vi "ad float to sample.vi"(6 "dbl":sgl, 7 "sample":u32, 8 "error in (no error)":errorcluster, 9 "range":i32, 10 "cha":i32, 11 "adh":i32) -> (0 "error out":errorcluster, 3 "function return":i32, 5 "sample out":u32)   [LabVIEW 2021, in "libad4.lvlib"]
doc: "ad_float_to_sample (int32_t adh, int32_t cha, int32_t range, float dbl, uint32_t *sample);\n\nConverts a float value into a sample value."
uses:
  <userlib>/libad4/libad4.lvlib
  <userlib>/libad4/libad4.dll
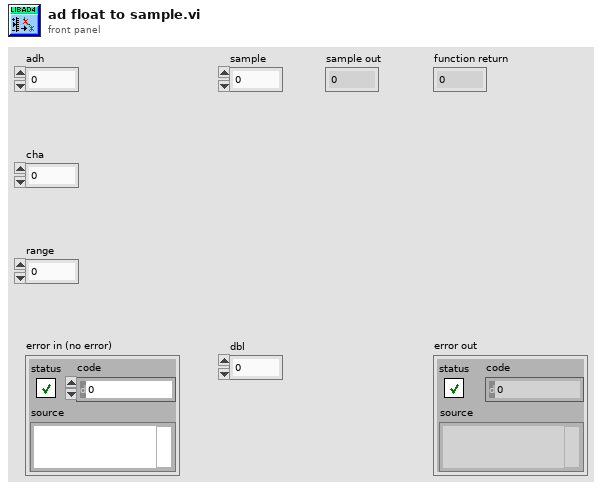
[diagram p1: front panel]
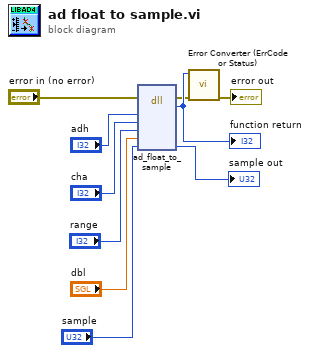
[diagram p0: block diagram]
diagram:
  n1 = dll-call lib="C:/Program Files/National Instruments/LabVIEW 2021/user.lib/libad4/libad4.*" fn="ad_float_to_sample"(error in="error in (no error)", "adh"="adh", "cha"="cha", "range"="range", "dbl"="dbl", "sample"="sample") -> (error out=w2:errorcluster, w10:i32, "sample"=→"sample out":u32)  [unwired: 6 in, 1 out]
  "function return" <- w10
  n2 = call <userlib>:"Error Converter (ErrCode or Status).vi"("error in (no error)"=w2, "error code"=w10) -> ("error out"=→"error out":errorcluster)  [unwired: 9 in]
